vi "AnalogToMiliVolts.vi"(10 "Input":dbl) -> (2 "Output":dbl)   [LabVIEW 2014]
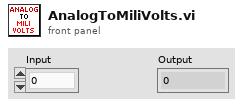
[diagram p1: front panel]
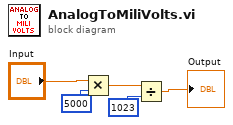
[diagram p0: block diagram]
diagram:
  n1 = Multiply(x="Input", y=5000) -> (x*y=w2:dbl)
  n2 = Divide(x=w2, y=1023) -> (x/y=→"Output":dbl)
